vi "xy_raster_scan.vi"(4 "Retract um":dbl format="%#_13g", 6 "YOffset um":dbl format="%#_13g", 7 "XOffset um":dbl format="%#_13g", 8 "YStepSize um":dbl format="%#_13g", 9 "XStepSize um":dbl format="%#_13g", 10 "YNum":i32, 11 "XNum":i32) -> (3 "Converted_HTT_Params":fxp<+/-,48,16>[](array[numeric]))   [LabVIEW 2024]
panel:
  out "appended array":dbl[][](array[numeric])
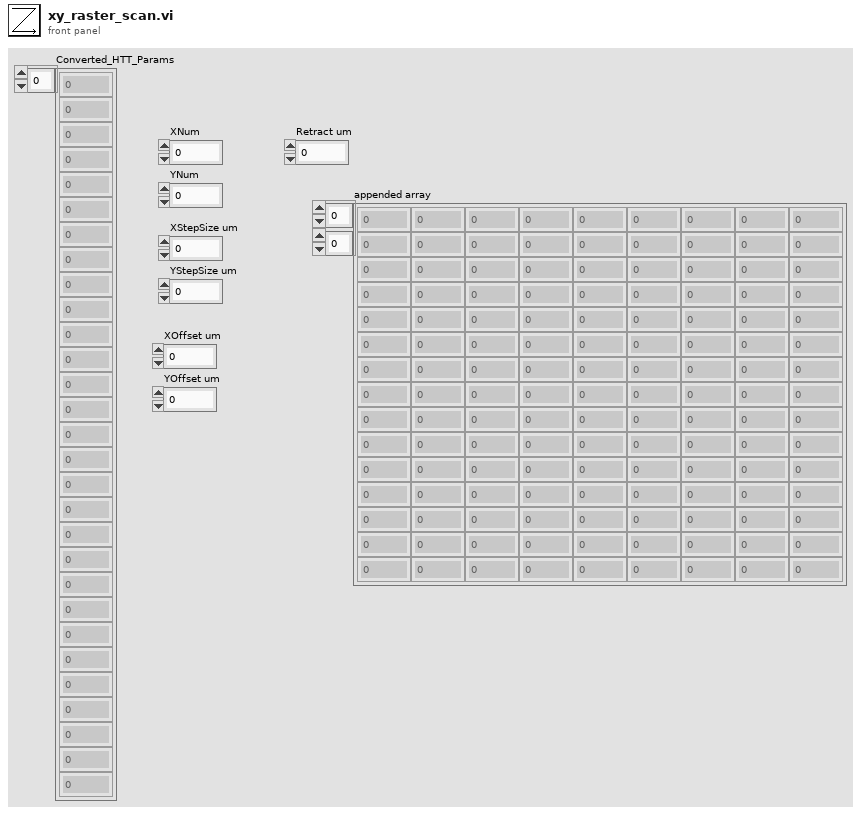
[diagram p1: front panel]
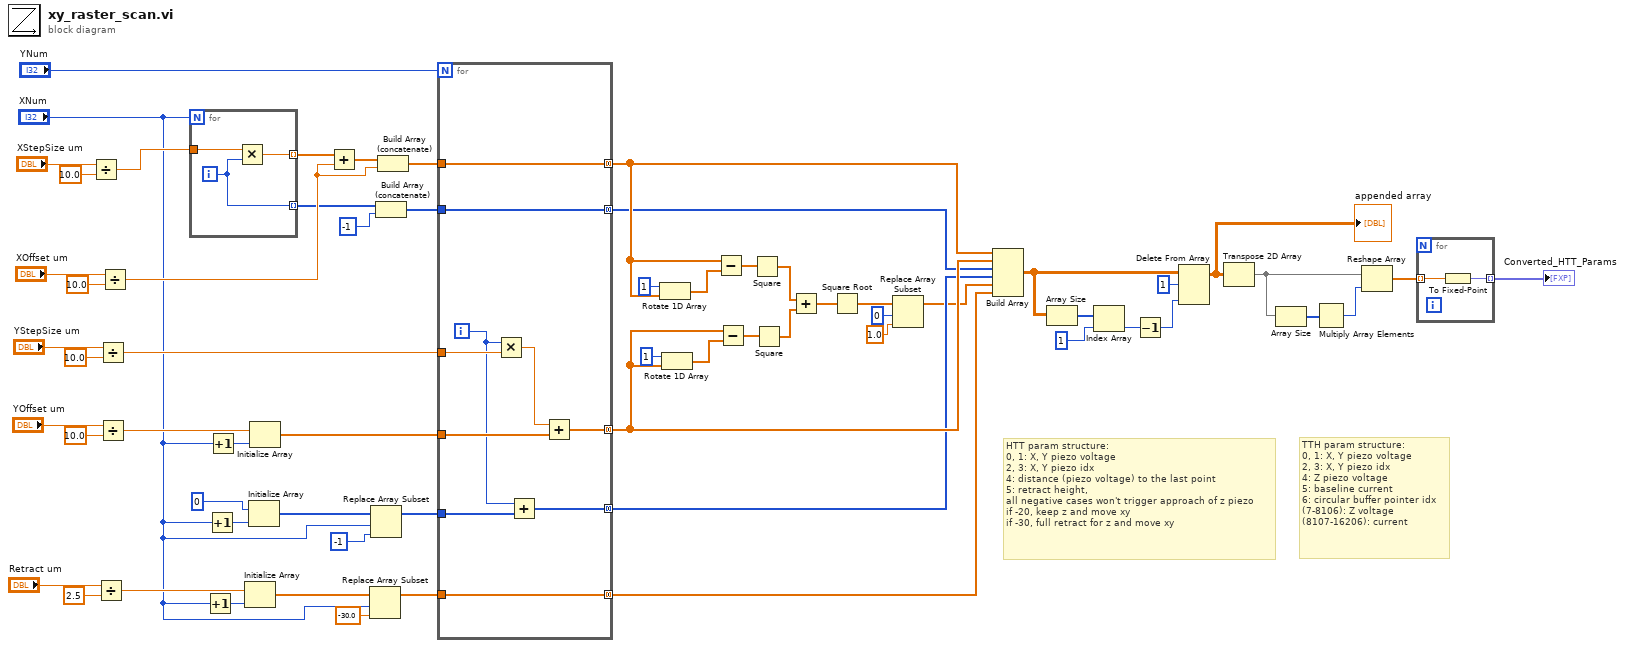
[diagram p0: block diagram]
diagram:
  # "TTH param structure:\n0, 1: X, Y piezo voltage\n2, 3: X, Y piezo idx\n4: Z piezo voltage\n5: baseline current\n6: circular buffer pointer idx\n(7-8106): Z voltage\n(8107-16206): current"
  # "HTT param structure:\n0, 1: X, Y piezo voltage\n2, 3: X, Y piezo idx\n4: distance (piezo voltage) to the last point\n5: retract height, \nall negative cases won't trigger approach of z piezo\nif -20, keep z and move xy\nif -30, full retract for z and move xy"
  n1 = Divide(x="XStepSize um", y=10.0) -> (x/y=w53:dbl)
  n2 = Divide(x="Retract um", y=2.5) -> (x/y=w40:dbl)
  n3 = Divide(x="YStepSize um", y=10.0) -> (x/y=w45:dbl)
  n4 = Divide(x="YOffset um", y=10.0) -> (x/y=w44:dbl)
  n5 = Divide(x="XOffset um", y=10.0) -> (x/y=w50:dbl)
  n6 = for {
    N: "XNum" -> [_]
    tunnel: w53 -> [w67]
    tunnel: [w66] -> w52 mode=indexing
    tunnel: [w65] -> w49 mode=indexing
    i -> [w65]
    n7 = Multiply(x=w67, y=w65) -> (x*y=w66:dbl)
  }
  n8 = Increment(x="XNum") -> (x+1=w41:i32)
  n9 = Increment(x="XNum") -> (x+1=w39:i32)
  n10 = Increment(x="XNum") -> (x+1=w43:i32)
  n11 = Initialize Array(w40, w41) -> (w20:dbl[])
  n12 = Initialize Array(0, w39) -> (w13:i32[])
  n13 = Initialize Array(w44, w43) -> (w42:dbl[])
  n14 = Add(x=w52, y=w50) -> (x+y=w51:dbl[])
  n15 = Replace Array Subset(array=w20, new element=-30.0 ("new element/subarray"), index="XNum") -> (w19:dbl[])
  n16 = Replace Array Subset(array=w13, new element=-1, index="XNum") -> (w12:i32[])
  n17 = Build Array (concatenate)(w49, -1) -> (w46:i32[])
  n18 = Build Array (concatenate)(w51, w50) -> (w47:dbl[])
  n19 = for {
    N: "YNum" -> [_]
    tunnel: w47 -> [w77]
    tunnel: w46 -> [w76]
    tunnel: [w77] -> w25 mode=concatenating
    tunnel: [w76] -> w23 mode=concatenating
    tunnel: w45 -> [w75]
    tunnel: w42 -> [w74]
    tunnel: [w72] -> w24 mode=concatenating
    tunnel: w19 -> [w71]
    tunnel: [w71] -> w16 mode=concatenating
    tunnel: w12 -> [w69]
    tunnel: [w68] -> w22 mode=concatenating
    i -> [w70]
    n20 = Multiply(x=w70, y=w75) -> (x*y=w73:dbl)
    n21 = Add(x=w70, y=w69) -> (x+y=w68:i32[])
    n22 = Add(x=w73, y=w74) -> (x+y=w72:dbl[])
  }
  n23 = Rotate 1D Array(1:w25, 2:1 ("n")) -> (0:w36:dbl[])
  n24 = Rotate 1D Array(1:w24, 2:1 ("n")) -> (0:w35:dbl[])
  n25 = Subtract(x=w25, y=w36) -> (x-y=w33:dbl[])
  n26 = Subtract(x=w24, y=w35) -> (x-y=w32:dbl[])
  n27 = Square(x=w33) -> (x^2=w31:dbl[])
  n28 = Square(x=w32) -> (x^2=w30:dbl[])
  n29 = Add(x=w31, y=w30) -> (x+y=w29:dbl[])
  n30 = Square Root(x=w29) -> (sqrt(x)=w28:dbl[])
  n31 = Replace Array Subset(array=w28, new element=1.0 ("new element/subarray"), index=0) -> (w21:dbl[])
  n32 = Build Array(w25, w24, w23, w22, w21, w16) -> (w7:dbl[][])
  n33 = Array Size(array=w7) -> (size(s)=w6:i32[])
  n34 = Index Array(array=w6, index=1) -> (element=w4:i32)
  n35 = Decrement(x=w4) -> (x-1=w3:i32)
  n36 = Delete From Array(array=w7, length=1, index (col)=w3) -> (array with subset deleted=w1:dbl[][])  [unwired: 1 in, 1 out]
  "appended array" <- w1
  n37 = Transpose 2D Array(2D array=w1) -> (transposed array=w2:dbl[][])
  n38 = Array Size(array=w2) -> (size(s)=w17:i32[])
  n39 = Multiply Array Elements(1:w17) -> (0:w8:i32)
  n40 = Reshape Array(w2, w8) -> (w15:dbl[])
  n41 = for {
    tunnel: w15 -> [w79] mode=indexing
    tunnel: [w78] -> w14 mode=indexing
    n42 = To Fixed-Point(number=w79) -> (fixed-point=w78:fxp<+/-,48,16>)  [unwired: 1 in]
  }
  "Converted_HTT_Params" <- w14
